vi "Read ResumeBlocked.vi"(8 "error in (no error)":errorcluster, 11 "GameMenu in":refnum<class "GameMenu.lvclass">) -> (0 "error out":errorcluster, 2 "ResumeBlocked":bool, 3 "GameMenu out":refnum<class "GameMenu.lvclass">)   [LabVIEW 2019, in "RT_Game.lvlib" / "GameMenu.lvclass"]
uses:
  GameMenu.lvclass
  GameMenu.lvclass/GameMenu.ctl
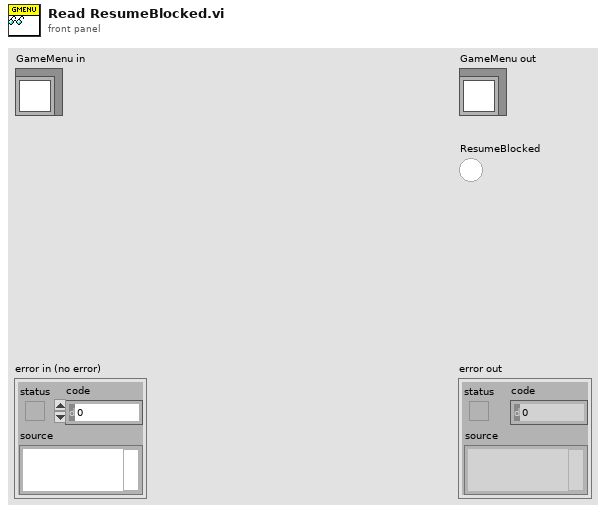
[diagram p1: front panel]
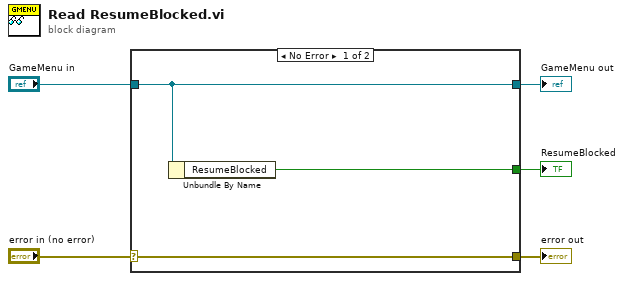
[diagram p0: block diagram]
diagram:
  n1 = case shown="No Error" "error in (no error)" {
    selector: "error in (no error)" -> [w8 w9]
    tunnel: [w8 w9] -> w4
    tunnel: [w7 w10] -> w2
    tunnel: "GameMenu in" -> [w7 w10]
    tunnel: [w6 _] -> w1
    frame No Error {
      n2 = Unbundle By Name(w7) -> ("ResumeBlocked"=w6:bool)
    }
    frame Error {
    }
  }
  "error out" <- w4
  "GameMenu out" <- w2
  "ResumeBlocked" <- w1
